vi "Vehicle Data.vi"(8 "error in":errorcluster, 9 "Logger In":refnum<queue>, 10 "Pipeline In":refnum<queue>, 11 "Vehicle Queue In":refnum<queue>) -> (0 "error out":errorcluster)   [LabVIEW 2016]
uses:
  Message Format.ctl
  StateDef_generic.ctl
  StateData_Vehicle.ctl
  <vilib>/addons/zeromq/socket_type.ctl
  <vilib>/addons/zeromq/socket_options.ctl
  <vilib>/addons/zeromq/zmq_context.lvclass
  <vilib>/addons/zeromq/zmq_socket.lvclass
  <vilib>/addons/zeromq/zeromq.lvlib
panel:
  out "Vehicle  Sensors":cluster{dbl, dbl, dbl}(graph)
  # "VEHICLE DATA"
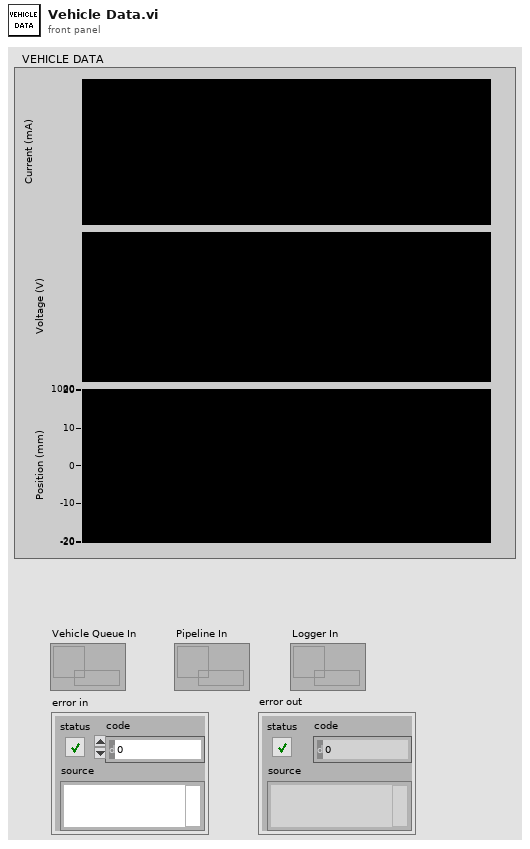
[diagram p1: front panel]
types:
  T1 = typedef "StateData_Vehicle.ctl" = cluster{"Current":dbl, "Voltage":dbl, "Position":dbl}
  T2 = typedef "StateDef_generic.ctl" = enum16{"Initialize", "Running", "Exit"}
  T3 = typedef "zeromq.lvlib/socket_options.ctl" = enum8{"NONE", "ZMQ_HWM", "<2>", "ZMQ_SWAP", "ZMQ_AFFINITY", "ZMQ_IDENTITY", "ZMQ_SUBSCRIBE", "ZMQ_UNSUBSCRIBE", "ZMQ_RATE", "ZMQ_RECOVERY_IVL", "ZMQ_MCAST_LOOP", "ZMQ_SNDBUF", "ZMQ_RCVBUF", "ZMQ_RCVMORE", "ZMQ_FD", "ZMQ_EVENTS", "ZMQ_TYPE", "ZMQ_LINGER", "ZMQ_RECONNECT_IVL", "ZMQ_BACKLOG", "ZMQ_RECOVERY_IVL_MSEC", "ZMQ_RECONNECT_IVL_MAX", "ZMQ_MAXMSGSIZE", "ZMQ_SNDHWM", "ZMQ_RCVHWM", "ZMQ_MULTICAST_HOPS", "<26>", "ZMQ_RCVTIMEO", "ZMQ_SNDTIMEO", "<29>", "<30>", "ZMQ_IPV4ONLY", "ZMQ_LAST_ENDPOINT", "ZMQ_ROUTER_MANDATORY", "ZMQ_TCP_KEEPALIVE", "ZMQ_TCP_KEEPALIVE_CNT", "ZMQ_TCP_KEEPALIVE_IDLE", "ZMQ_TCP_KEEPALIVE_INTVL", "ZMQ_TCP_ACCEPT_FILTER", "ZMQ_DELAY_ATTACH_ON_CONNECT", "ZMQ_XPUB_VERBOSE"}
  T4 = typedef "zeromq.lvlib/socket_type.ctl" = enum8{"ZMQ_PAIR", "ZMQ_PUB", "ZMQ_SUB", "ZMQ_REQ", "ZMQ_REP", "ZMQ_DEALER", "ZMQ_ROUTER", "ZMQ_PULL", "ZMQ_PUSH", "ZMQ_XPUB", "ZMQ_XSUB"}
  T5 = typedef "Message Format.ctl" = cluster{"header":string, "data":variant}
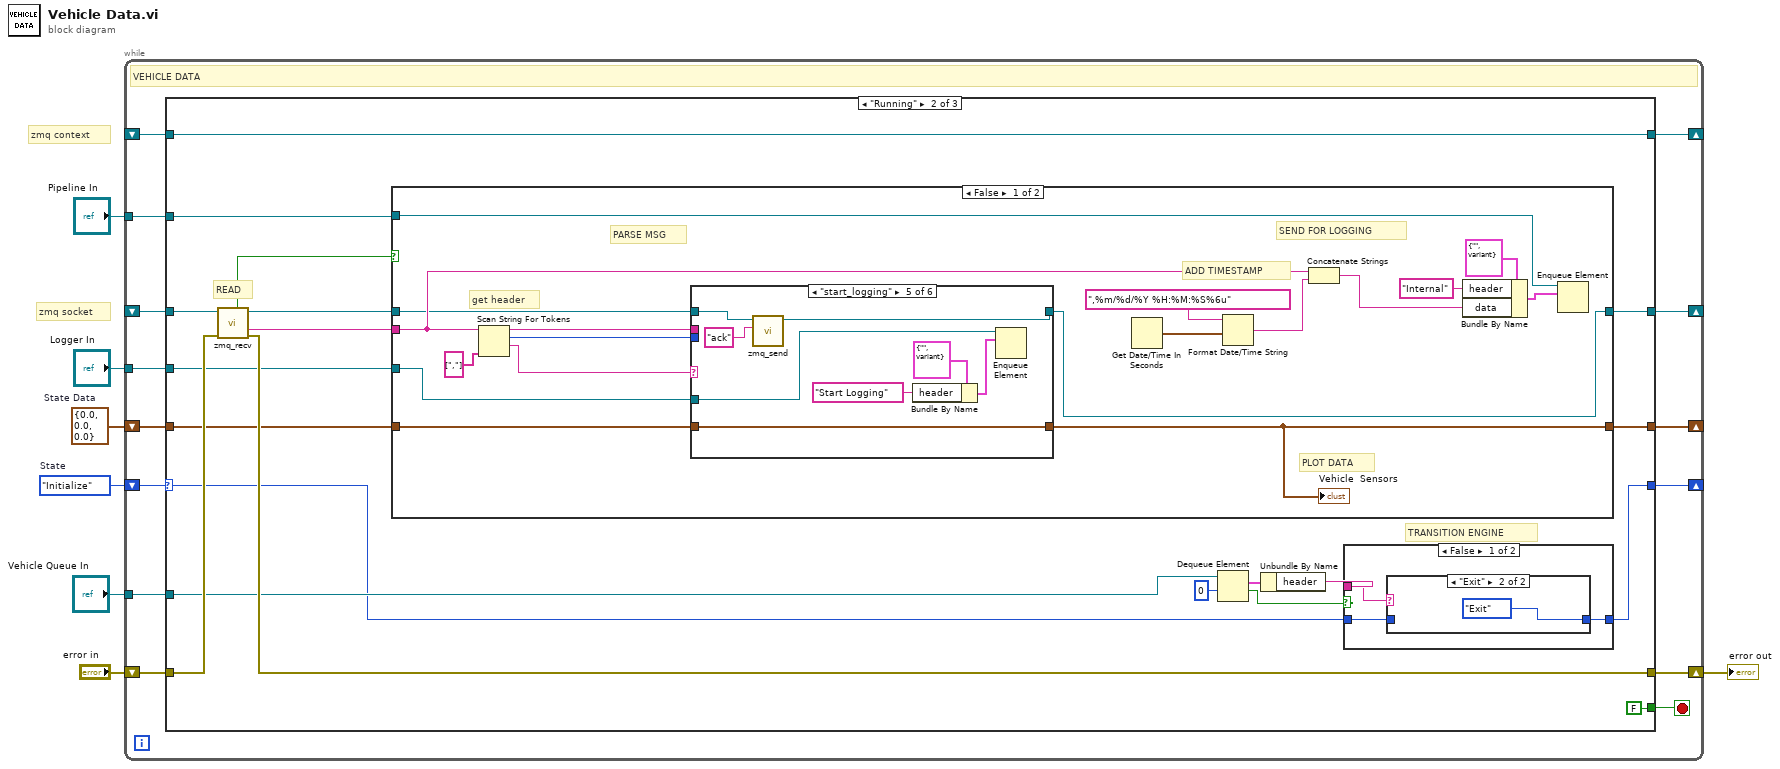
[diagram p0: block diagram]
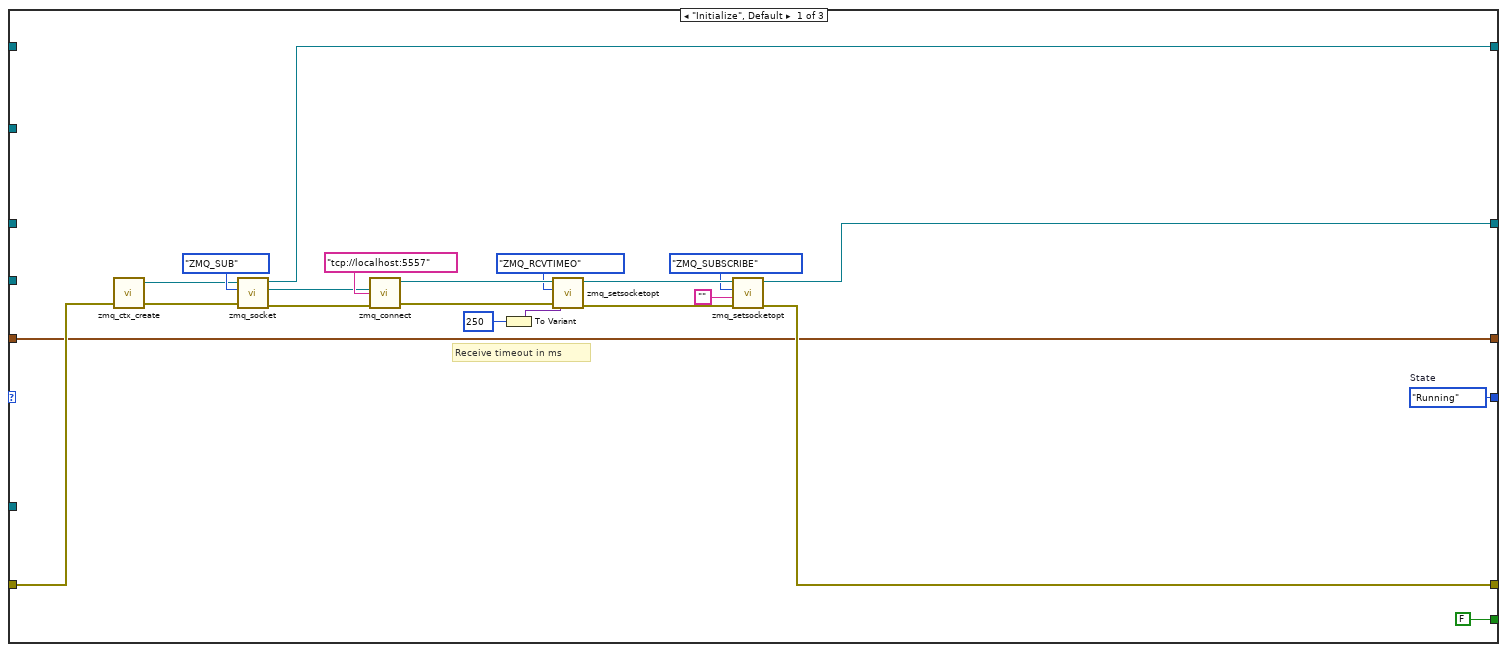
[diagram p2: hidden frame]
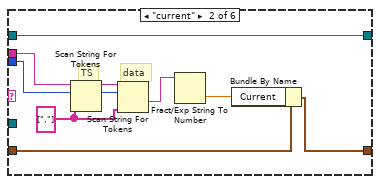
[diagram p6: hidden frame]
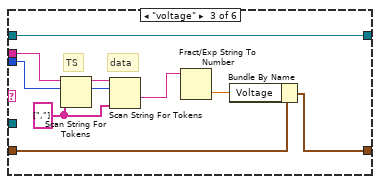
[diagram p7: hidden frame]
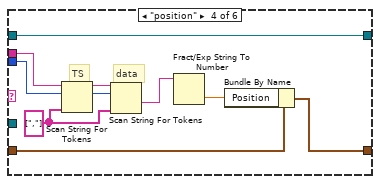
[diagram p8: hidden frame]
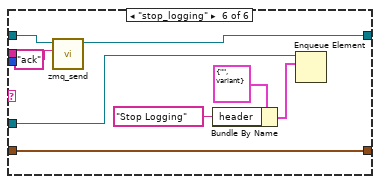
[diagram p9: hidden frame]
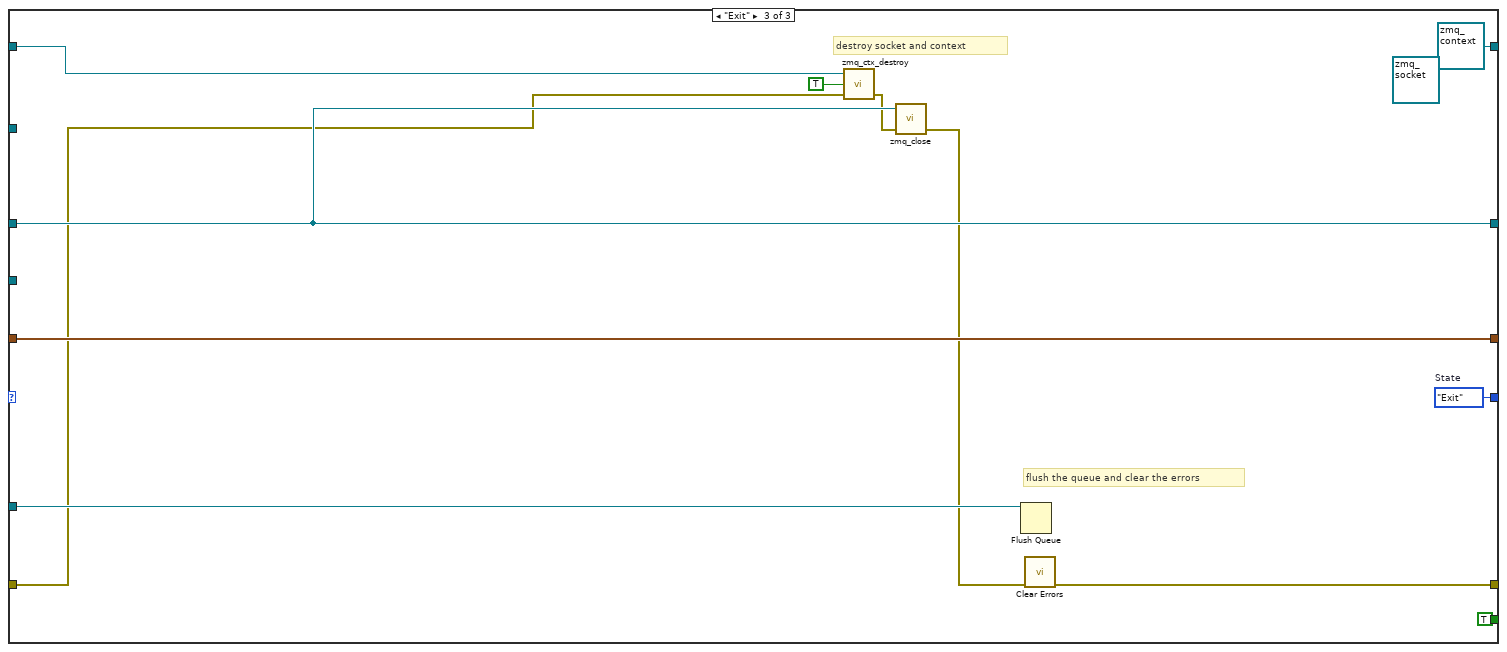
[diagram p11: hidden frame]
diagram:
  w2 = T1 {"Current"=0.0, "Voltage"=0.0, "Position"=0.0}  # State Data
  w4 = StateDef_generic."Initialize"  # State
  # "zmq socket"
  # "zmq context"
  n1 = while {
    shift-right: [w21] -> w3
    shift-left: "error in" -> [w16]
    shift-right: [w8] -> _
    shift-left: _ -> [w20]
    shift-right: [w19] -> _
    shift-left: _ -> [w18]
    tunnel: "Pipeline In" -> [w14]
    tunnel: "Vehicle Queue In" -> [w15]
    shift-right: [w12] -> _
    shift-left: w4 -> [w17]
    shift-right: [w10] -> _
    shift-left: w2 -> [w11]
    tunnel: "Logger In" -> [w9]
    stop <- w13 stop-if-true
    # "VEHICLE DATA"
    n2 = case shown="\"Running\"" w17 {
      selector: w17 -> [_ w48 _]
      tunnel: [w26 w61 w140] -> w21
      tunnel: w20 -> [_ w62 w148]
      tunnel: [w30 w63 refnum<class "zmq_context.lvclass"> refnum ("context out")] -> w19
      tunnel: w18 -> [_ w63 w149]
      tunnel: w16 -> [w27 w59 w139]
      tunnel: w15 -> [_ w50 w143]
      tunnel: w14 -> [_ w55 _]
      tunnel: [FALSE FALSE TRUE] -> w13
      tunnel: [w24 w44 w145] -> w12
      tunnel: w11 -> [w23 w56 w144]
      tunnel: [w23 w54 w144] -> w10
      tunnel: w9 -> [_ w47 _]
      tunnel: [w22 w45 w148] -> w8
      frame "Initialize", Default {
        w24 = StateDef_generic."Running"  # State
        # "Receive timeout in ms"
        n3 = call <vilib>:"zmq_ctx_create.vi"("error in"=w27) -> ("error out"=w36:errorcluster, "context out"=w35:refnum<class "zmq_context.lvclass">)  [unwired: 3 in]
        n4 = call <vilib>:"zmq_socket.vi"("error in"=w36, "socket type"=socket_type."ZMQ_SUB", "context in"=w35) -> ("error out"=w39:errorcluster, "socket out"=w38:refnum<class "zmq_socket.lvclass">, "context out"=w30:refnum<class "zmq_context.lvclass">)  [unwired: 2 in]
        n5 = call <vilib>:"zmq_connect.vi"("error in"=w39, "endpoint"="tcp://localhost:5557", "socket in"=w38) -> ("error out"=w43:errorcluster, "socket out"=w42:refnum<class "zmq_socket.lvclass">)  [unwired: 1 in]
        n6 = To Variant(anything=250) -> (Variant=w28:variant)
        n7 = call <vilib>:"zmq_setsocketopt.vi"("error in"=w43, "value"=w28, "option"=socket_options."ZMQ_RCVTIMEO", "socket in"=w42) -> ("error out"=w33:errorcluster, "socket out"=w34:refnum<class "zmq_socket.lvclass">)  [unwired: 2 in]
        n8 = call <vilib>:"zmq_setsocketopt.vi"("error in"=w33, "value"="", "option"=socket_options."ZMQ_SUBSCRIBE", "socket in"=w34) -> ("error out"=w26:errorcluster, "socket out"=w22:refnum<class "zmq_socket.lvclass">)  [unwired: 2 in]
      }
      frame "Running" {
        # "TRANSITION ENGINE"
        # "READ"
        n9 = call <vilib>:"zmq_recv.vi"("error in"=w59, "socket in"=w62) -> ("error out"=w61:errorcluster, "data"=w57:string, "socket out"=w46:refnum<class "zmq_socket.lvclass">, "timeout?"=w60:bool)  [unwired: 3 in, 1 out]
        n10 = case shown="False" w60 {
          tunnel: w57 -> [w80 _]
          tunnel: w56 -> [w78 w137]
          tunnel: [w77 w137] -> w54
          tunnel: w55 -> [w76 _]
          tunnel: w47 -> [w73 _]
          tunnel: w46 -> [w72 w136]
          tunnel: [w71 w136] -> w45
          frame False {
            # "ADD TIMESTAMP"
            # "SEND FOR LOGGING"
            # "PLOT DATA"
            # "PARSE MSG"
            # "get header"
            n11 = Scan String For Tokens(6:string[] [","], 9:w80) -> (1:w75:string, 2:w70:i32, 3:w74:string)  [unwired: 4 in, 1 out]
            n12 = case shown="\"start_logging\"" w75 {
              tunnel: [w89 w98 w108 w118 w127 w135] -> w77
              tunnel: w78 -> [w89 w99 w109 w119 w127 w135]
              tunnel: w74 -> [_ w95 w103 w115 _ _]
              tunnel: w73 -> [_ _ _ _ w126 w134]
              tunnel: w72 -> [w88 w93 w104 w114 w121 w130]
              tunnel: [w88 w93 w104 w114 w120 w128] -> w71
              tunnel: w70 -> [_ w91 w101 w111 _ _]
              frame "other", Default {
              }
              frame "current" {
                w92 = string[] [","]
                # "data"
                # "TS"
                n13 = Scan String For Tokens(6:w92, 8:w91, 9:w95) -> (2:w90:i32, 3:w97:string)  [unwired: 3 in, 2 out]
                n14 = Scan String For Tokens(6:w92, 8:w90, 9:w97) -> (1:w96:string)  [unwired: 3 in, 3 out]
                n15 = Fract/Exp String To Number(string=w96) -> (number=w94:dbl)  [unwired: 3 in, 1 out]
                n16 = Bundle By Name(cluster=w99, "Current"=w94) -> (w98:T1)
              }
              frame "voltage" {
                w102 = string[] [","]
                # "data"
                # "TS"
                n17 = Scan String For Tokens(6:w102, 8:w101, 9:w103) -> (2:w100:i32, 3:w107:string)  [unwired: 3 in, 2 out]
                n18 = Scan String For Tokens(6:w102, 8:w100, 9:w107) -> (1:w106:string)  [unwired: 3 in, 3 out]
                n19 = Fract/Exp String To Number(string=w106) -> (number=w105:dbl)  [unwired: 3 in, 1 out]
                n20 = Bundle By Name(cluster=w109, "Voltage"=w105) -> (w108:T1)
              }
              frame "position" {
                w113 = string[] [","]
                # "data"
                # "TS"
                n21 = Scan String For Tokens(6:w113, 8:w111, 9:w115) -> (2:w110:i32, 3:w117:string)  [unwired: 3 in, 2 out]
                n22 = Scan String For Tokens(6:w113, 8:w110, 9:w117) -> (1:w116:string)  [unwired: 3 in, 3 out]
                n23 = Fract/Exp String To Number(string=w116) -> (number=w112:dbl)  [unwired: 3 in, 1 out]
                n24 = Bundle By Name(cluster=w119, "Position"=w112) -> (w118:T1)
              }
              frame "start_logging" {
                n25 = call <vilib>:"zmq_send.vi"("data"="ack", "socket in"=w121) -> ("socket out"=w120:refnum<class "zmq_socket.lvclass">)  [unwired: 5 in, 1 out]
                n26 = Bundle By Name(cluster=T5 {"header"="", "data"=variant} ("msg format"), "header"="Start Logging") -> (w123:T5)
                n27 = Enqueue Element(queue=w126, element=w123) -> ()  [unwired: 2 in, 3 out]
              }
              frame "stop_logging" {
                n28 = call <vilib>:"zmq_send.vi"("data"="ack", "socket in"=w130) -> ("socket out"=w128:refnum<class "zmq_socket.lvclass">)  [unwired: 5 in, 1 out]
                n29 = Bundle By Name(cluster=T5 {"header"="", "data"=variant} ("msg format"), "header"="Stop Logging") -> (w131:T5)
                n30 = Enqueue Element(queue=w134, element=w131) -> ()  [unwired: 2 in, 3 out]
              }
            }
            "Vehicle  Sensors" <- w77
            n31 = Get Date/Time In Seconds() -> (seconds since 1Jan1904=w83:timestamp)
            n32 = Format Date/Time String(time format string (%c)=",%m/%d/%Y %H:%M:%S%6u", seconds (now)=w83) -> (date/time string=w81:string)  [unwired: 1 in]
            n33 = Concatenate Strings(w80, w81) -> (w79:string)
            n34 = Bundle By Name(cluster=T5 {"header"="", "data"=variant} ("msg format"), "header"="Internal", "data"=w79) -> (w84:T5)
            n35 = Enqueue Element(queue=w76, element=w84) -> ()  [unwired: 2 in, 3 out]
          }
          frame True {
          }
        }
        n36 = Dequeue Element(queue=w50, timeout in ms (-1)=0) -> (element=w52:T5, timed out?=w49:bool)  [unwired: 1 in, 2 out]
        n37 = Unbundle By Name(w52) -> ("header"=w51:string)
        n38 = case shown="False" w49 {
          tunnel: w51 -> [w66 _]
          tunnel: [w65 w69] -> w44
          tunnel: w48 -> [w64 w69]
          frame False {
            n39 = case shown="\"Exit\"" w66 {
              tunnel: [w67 StateDef_generic."Exit" ("State")] -> w65
              tunnel: w64 -> [w67 _]
              frame "any other", Default {
              }
              frame "Exit" {
              }
            }
          }
          frame True {
          }
        }
      }
      frame "Exit" {
        (unwired) refnum<class "zmq_socket.lvclass"> refnum ("socket out")
        w145 = StateDef_generic."Exit"  # State
        # "destroy socket and context"
        # "flush the queue and clear the errors"
        n40 = call <vilib>:"zmq_ctx_destroy.vi"("error in"=w139, "reap? (F)"=TRUE, "context in"=w149) -> ("error out"=w141:errorcluster)  [unwired: 2 in]
        n41 = call <vilib>:"zmq_close.vi"("error in"=w141, "socket"=w148) -> ("error out"=w138:errorcluster)  [unwired: 3 in]
        n42 = Flush Queue(queue=w143) -> ()  [unwired: 1 in, 3 out]
        n43 = call <vilib>:"Clear Errors.vi"("error in (no error)"=w138) -> ("error out"=w140:errorcluster)  [unwired: 5 in, 1 out]
      }
    }
  }
  "error out" <- w3
